vi "Read CtlRef.vi"(8 "error in (no error)":errorcluster, 11 "ShortcutMenuSelectionMsg in":refnum<class "ShortcutMenuSelectionMsg.lvclass">) -> (0 "error out":errorcluster, 2 "CtlRef":refnum<vi>, 3 "ShortcutMenuSelectionMsg out":refnum<class "ShortcutMenuSelectionMsg.lvclass">)   [LabVIEW 2017, in "ActorEvents.lvlib" / "ShortcutMenuSelectionMsg.lvclass"]
uses:
  ShortcutMenuSelectionMsg.lvclass
  ShortcutMenuSelectionMsg.lvclass/ShortcutMenuSelectionMsg.ctl
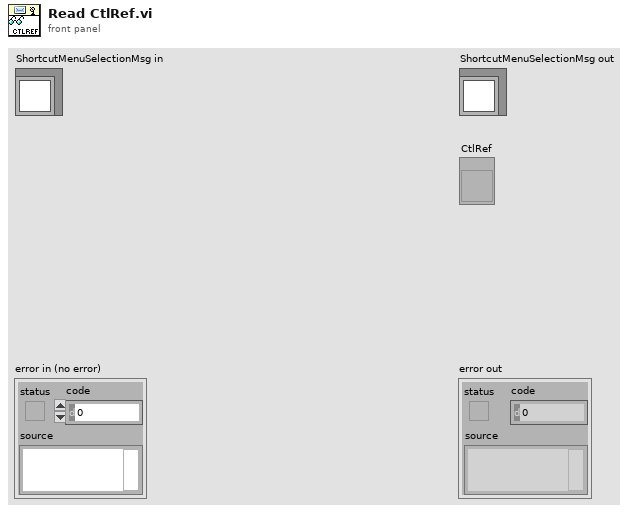
[diagram p1: front panel]
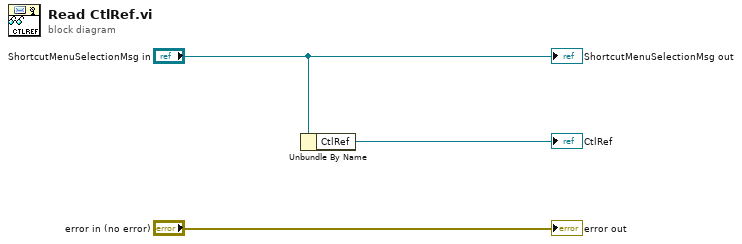
[diagram p0: block diagram]
diagram:
  n1 = Unbundle By Name("ShortcutMenuSelectionMsg in") -> ("CtlRef"=→"CtlRef":refnum<vi>)
  "error out" <- "error in (no error)"
  "ShortcutMenuSelectionMsg out" <- "ShortcutMenuSelectionMsg in"
